vi "Actor Loop.vi"(11 "Actor in":refnum<class "Actor.lvclass">) -> ()   [LabVIEW 2021, in "jettl.lvlib" / "Actor.lvclass"]
uses:
  Actor.lvclass
  Msg Strategy/Msg Strategy.lvclass
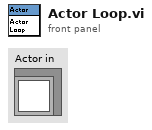
[diagram p1: front panel]
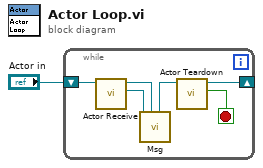
[diagram p0: block diagram]
diagram:
  n1 = while {
    shift-right: [w7] -> _
    shift-left: "Actor in" -> [w4]
    stop <- w5 stop-if-true
    n2 = call-dynamic "Actor Receive.vi"("Actor in"=w4) -> ("Msg"=w6:refnum<class "Msg Strategy.lvclass">, "Actor out"=w3:refnum<class "Actor.lvclass">)  [unwired: 9 in]
    n3 = call-dynamic "Msg.vi"("Actor in"=w3, "Msg Strategy in"=w6) -> ("Actor out"=w2:refnum<class "Actor.lvclass">)  [unwired: 9 in]
    n4 = call-dynamic "Actor Teardown.vi"("Actor in"=w2) -> ("Teardown?"=w5:bool, "Actor out"=w7:refnum<class "Actor.lvclass">)  [unwired: 9 in]
  }
